vi "Generate Data.vi"(8 "에러 입력":errorcluster caption="에러 입력(에러 없음)", 11 "채널 수":i32) -> (0 "에러 출력":errorcluster, 2 "파워 스펙트럼 데이터":waveform(dbl)[](graph) caption="파워 스펙트럼", 3 "웨이브폼 차트":waveform(dbl)[](graph))   [LabVIEW 2010]
uses:
  <vilib>/express/express analysis/Spectral/XNode/ExpressSpectralMeasurementsBlockNode.xnode
  Instance           3 21Saved   Generate Data .vi
  Instance           4 21Saved   Generate Data .vi
  Instance           1 21Saved   Generate Data .vi
  <vilib>/express/express analysis/Spectral/Block/exnSpectralBlock spectral measurements power poly.vi
  <vilib>/express/express analysis/Spectral/Block/exnSpectralBlock spectral measurements power DDT.vi
panel:
  in  "공백":dynamicdata(waveform)
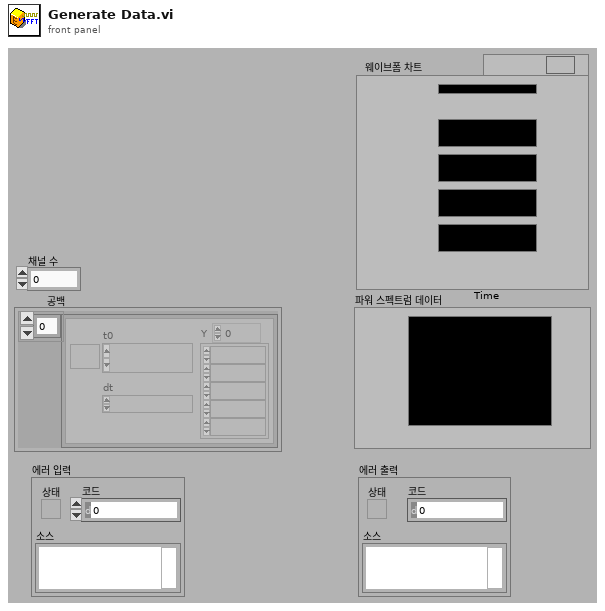
[diagram p1: front panel]
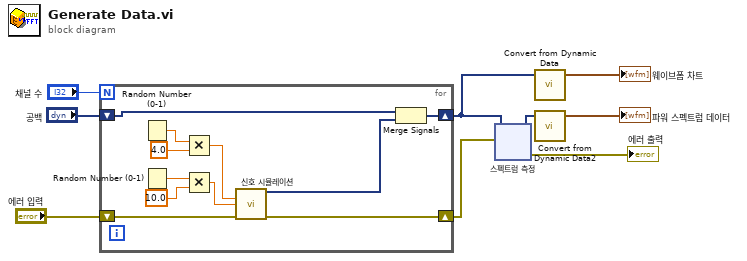
[diagram p0: block diagram]
diagram:
  n1 = for {
    N: "채널 수" -> [_]
    shift-right: [w13] -> w8
    shift-left: "에러 입력" -> [w17]
    shift-right: [w16] -> w6
    shift-left: "공백" -> [w14]
    n2 = Random Number (0-1)() -> (number: 0 to 1=w11:dbl)
    n3 = Random Number (0-1)() -> (number: 0 to 1=w20:dbl)
    n4 = Multiply(x=w11, y=4.0) -> (x*y=w10:dbl)
    n5 = Multiply(x=w20, y=10.0) -> (x*y=w18:dbl)
    n6 = call "신호 시뮬레이션"("Frequency"=w10, "Amplitude"=w18, "error in (no error)"=w17) -> ("Sine"=w15:dynamicdata, "error out"=w13:errorcluster)  [unwired: 11 in]
    n7 = Merge Signals(w14, w15) -> (w16:dynamicdata)
  }
  n8 = xnode "스펙트럼 측정"("신호"=w6, "에러 입력(에러 없음)"=w8) -> ("Power Spectrum"=w4:dynamicdata, "에러 출력"=→"에러 출력":errorcluster)
  n9 = call "Convert from Dynamic Data"("Dynamic Data Type"=w6) -> ("Array of Waveform"=→"웨이브폼 차트":waveform(dbl)[])  [unwired: 3 in]
  n10 = call "Convert from Dynamic Data2"("Dynamic Data Type"=w4) -> ("Array of Waveform"=→"파워 스펙트럼 데이터":waveform(dbl)[])  [unwired: 3 in]
